vi "Determine Next Operation.vi"(0 "Initialize Array in":bool[](array[boolean]), 1 "Record Array in":T1[](array[typedef]), 5 "Processed Calibration Point":T1, 7 "Test Parameters":T4 {"Allowed Tolerance (%) FS" format="%#_4g"}, 9 "Array in":waveform(dbl)[](array[waveform]), 11 "error in (no error)":errorcluster, 12 "Array Index or Channel":i32) -> (3 "Record Array out":T1[](array[typedef]), 4 "Initialize Array out":bool[](array[boolean]), 6 "Record?":bool, 8 "Done?":bool, 10 "Recorded Channels":bool[](array[boolean]), 15 "error out":errorcluster)   [LabVIEW 2026, in "Processing_Engine.lvlib"]
uses:
  Processing_Engine.lvlib
  Test Parameters Cluster.ctl
  controls/Messaging Payloads/Processed Calibration Point.ctl
  controls/UI/Direction.ctl
  Test Status.ctl
  Settings/Settings.lvlib
  Analysis/Analysis.lvlib
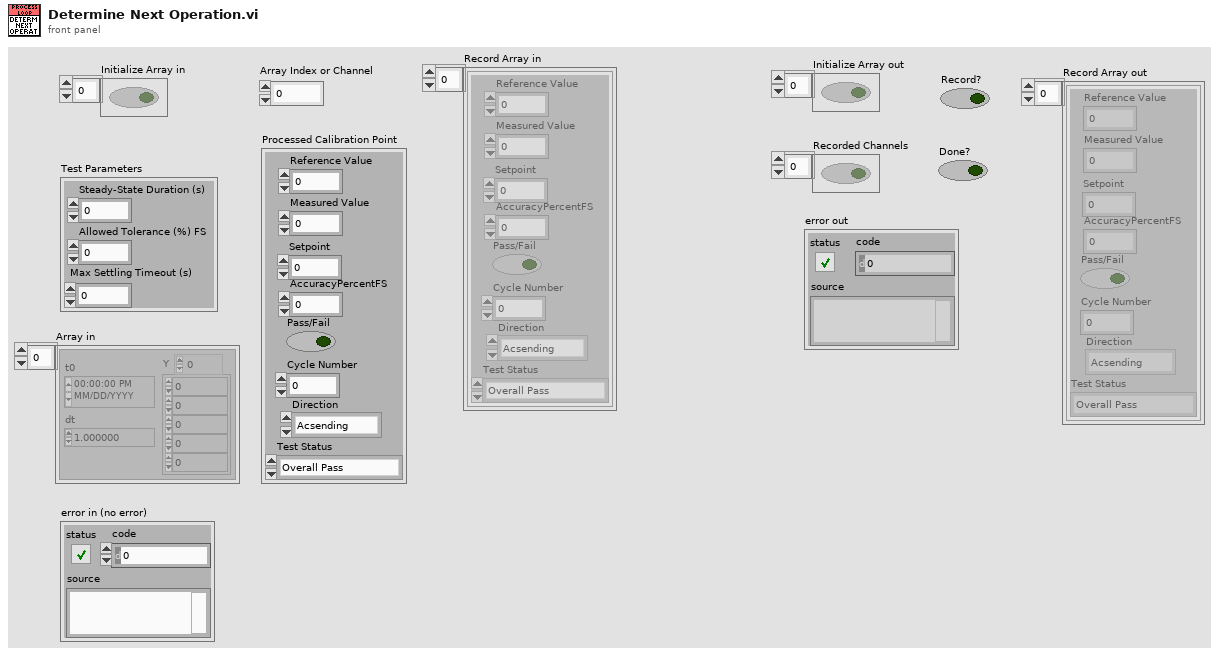
[diagram p1: front panel]
types:
  T1 = typedef "Processed Calibration Point.ctl" = cluster{"Reference Value":dbl, "Measured Value":dbl, "AccuracyPercentFS":dbl, "Pass/Fail":bool, "Setpoint":dbl, "Cycle Number":i32, "Direction":T2, "Test Status":T3}
  T2 = typedef "Settings.lvlib/Direction.ctl" = enum16{"Acsending", "Descending"}
  T3 = typedef "Analysis.lvlib/Test Status.ctl" = enum16{"Overall Pass", "Overall Fail", "Test Running"}
  T4 = typedef "Settings.lvlib/Test Parameters Cluster.ctl" = cluster{"Steady-State Duration (s)":i32, "Allowed Tolerance (%) FS":dbl, "Max Settling Timeout (s)":i32}
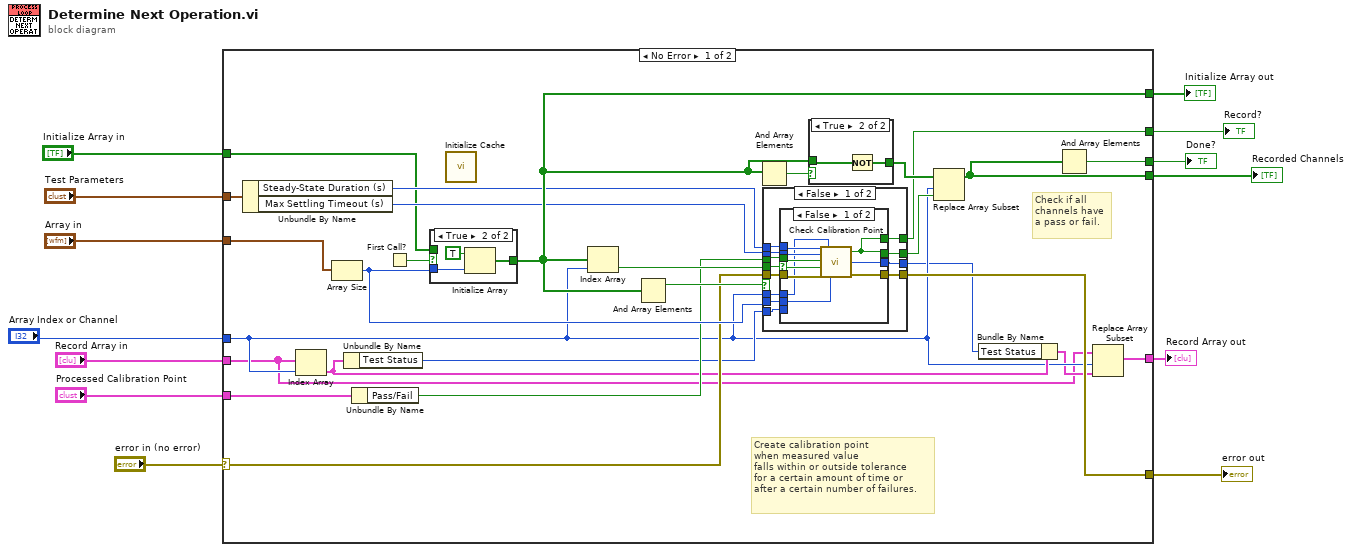
[diagram p0: block diagram]
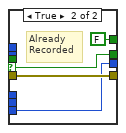
[diagram p3: hidden frame]
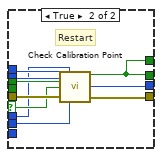
[diagram p4: hidden frame]
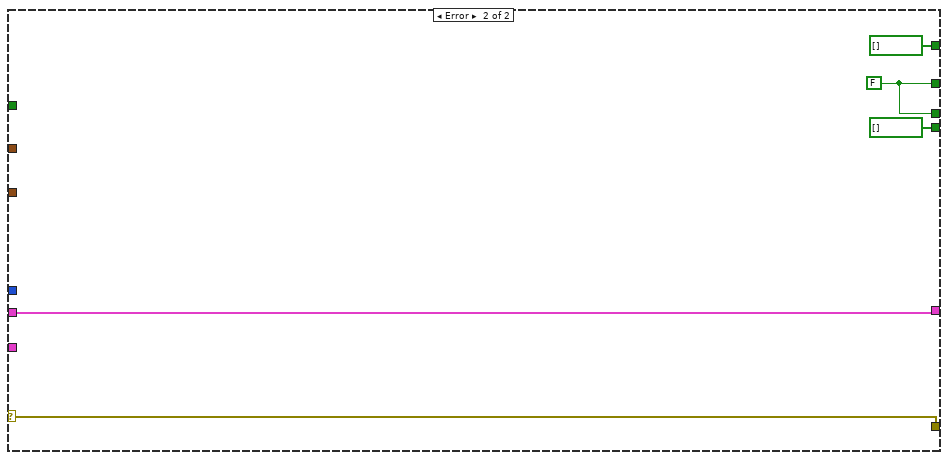
[diagram p6: hidden frame]
diagram:
  n1 = case shown="No Error" "error in (no error)" {
    selector: "error in (no error)" -> [w22 w85]
    tunnel: "Array in" -> [w40 _]
    tunnel: [w38 bool[] [] ("Initialize Array in")] -> w12
    tunnel: "Array Index or Channel" -> [w18 _]
    tunnel: [w35 w85] -> w10
    tunnel: [w34 w87] -> w9
    tunnel: [w31 w87] -> w8
    tunnel: "Initialize Array in" -> [w27 _]
    tunnel: [w25 bool[] [] ("Initialize Array in")] -> w6
    tunnel: "Test Parameters" -> [w24 _]
    tunnel: "Processed Calibration Point" -> [w21 _]
    tunnel: "Record Array in" -> [w15 w84]
    tunnel: [w16 w84] -> w1
    frame No Error {
      # "Create calibration point\nwhen measured value\nfalls within or outside tolerance\nfor a certain amount of time or \nafter a certain number of failures."
      # "Check if all\nchannels have\na pass or fail."
      n2 = Unbundle By Name(w24) -> ("Steady-State Duration (s)"=w33:i32, "Max Settling Timeout (s)"=w32:i32)
      n3 = Index Array(array=w15, index=w18) -> (element=w19:T1)
      n4 = Array Size(array=w40) -> (size(s)=w36:i32)
      n5 = Unbundle By Name(w19) -> ("Test Status"=w20:T3)
      n6 = Unbundle By Name(w21) -> ("Pass/Fail"=w23:bool)
      n7 = First Call?() -> (First Call?: T/F=w26:bool)
      n8 = case shown="True" w26 {
        tunnel: w36 -> [_ w82]
        tunnel: [w80 w81] -> w38
        tunnel: w27 -> [w80 _]
        frame False {
        }
        frame True {
          n9 = Initialize Array(TRUE ("Record?"), w82) -> (w81:bool[])
        }
      }
      n10 = call "Initialize Cache.vi"() -> ()  [unwired: 10 in, 2 out]
      n11 = Index Array(array=w38, index=w18) -> (element=w28:bool)
      n12 = And Array Elements(Boolean array=w38) -> (logical AND=w29:bool)
      n13 = And Array Elements(Boolean array=w38) -> (logical AND=w37:bool)
      n14 = case shown="False" w29 {
        selector: w29 -> [_ w73]
        tunnel: w22 -> [w55 w79]
        tunnel: [w54 w78] -> w35
        tunnel: [w53 w74] -> w30
        tunnel: w23 -> [w52 w77]
        tunnel: w28 -> [w51 _]
        tunnel: w32 -> [w50 w76]
        tunnel: w33 -> [w49 w75]
        tunnel: [w48 w74] -> w34
        tunnel: w18 -> [w47 w72]
        tunnel: w36 -> [w46 w71]
        tunnel: [w45 w70] -> w14
        tunnel: w20 -> [w44 _]
        frame False {
          n15 = case shown="False" w51 {
            selector: w51 -> [w62 w68]
            tunnel: w55 -> [w65 w69]
            tunnel: [w64 w69] -> w54
            tunnel: [w59 w68] -> w53
            tunnel: w52 -> [w63 _]
            tunnel: w50 -> [w61 _]
            tunnel: w49 -> [w60 _]
            tunnel: [w59 FALSE] -> w48
            tunnel: w47 -> [w58 _]
            tunnel: w46 -> [w57 _]
            tunnel: [w56 w66] -> w45
            tunnel: w44 -> [_ w66]
            frame False {
              n16 = call "Check Calibration Point.vi"("Steady State Duration"=w60, "Channel"=w58, "Maximum Settling Timeout"=w61, "Pass Flag?"=w63, "Reset?"=w62, "error in (no error)"=w65, "Number of Channels"=w57) -> ("Record?"=w59:bool, "Test Status"=w56:T3, "error out"=w64:errorcluster)  [unwired: 6 in]
            }
            frame True {
              # "Already\nRecorded"
            }
          }
        }
        frame True {
          # "Restart"
          n17 = call "Check Calibration Point.vi"("Steady State Duration"=w75, "Channel"=w72, "Maximum Settling Timeout"=w76, "Pass Flag?"=w77, "Reset?"=w73, "error in (no error)"=w79, "Number of Channels"=w71) -> ("Record?"=w74:bool, "Test Status"=w70:T3, "error out"=w78:errorcluster)  [unwired: 6 in]
        }
      }
      n18 = case shown="True" w37 {
        tunnel: w38 -> [w41 w43]
        tunnel: [w41 w42] -> w39
        frame False {
        }
        frame True {
          n19 = Not(x=w43) -> (.not. x?=w42:bool[])
        }
      }
      n20 = Replace Array Subset(array=w39, new element=w30, index=w18) -> (w25:bool[])
      n21 = Bundle By Name(cluster=w19, "Test Status"=w14) -> (w17:T1)
      n22 = And Array Elements(Boolean array=w25) -> (logical AND=w31:bool)
      n23 = Replace Array Subset(array=w15, new element=w17, index=w18) -> (w16:T1[])
    }
    frame Error {
      w87 = FALSE ("Record?")
    }
  }
  "Initialize Array out" <- w12
  "error out" <- w10
  "Record?" <- w9
  "Done?" <- w8
  "Recorded Channels" <- w6
  "Record Array out" <- w1
